vi "MotorSpeedv3.vi"(6 "MotrSpdInfo":T1={"TrgtCounts"=0, "Accel?"=FALSE, "CurrCounts"=0.0, "SlowRng"=572.75, "MinPwr"=572.75} {"MinPwr" format="%#_13g"; "SlowRng" format="%#_13g"}, 7 "MaxPwr":dbl, 8 "RightSpdIn":dbl, 10 "FirstTime?":bool, 11 "LeftSpdIn":dbl) -> (0 "RightSpdOut":dbl, 3 "LeftSpdOut":dbl)   [LabVIEW 2017]
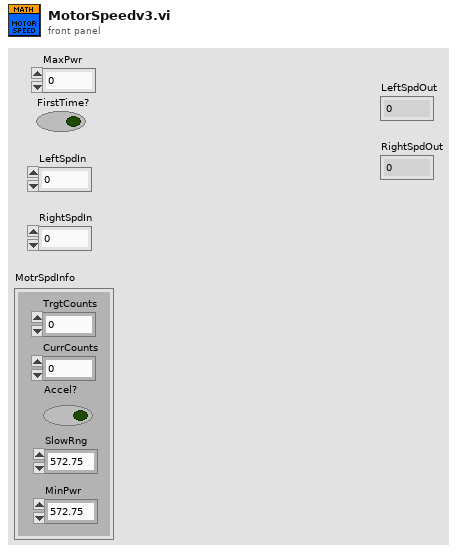
[diagram p1: front panel]
types:
  T1 = cluster{"TrgtCounts":i32, "Accel?":bool, "CurrCounts":dbl, "SlowRng":dbl, "MinPwr":dbl}
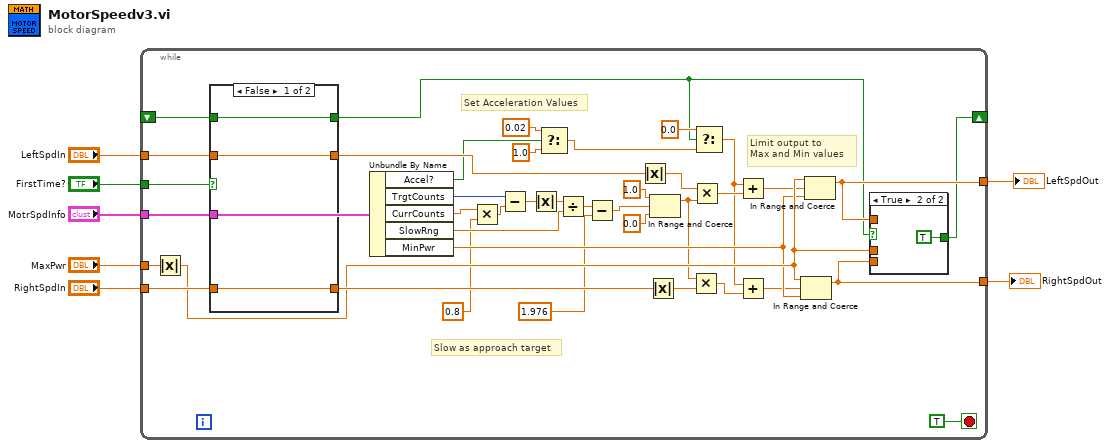
[diagram p0: block diagram]
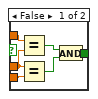
[diagram p2: hidden frame]
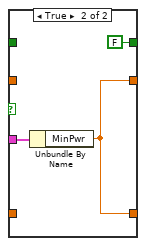
[diagram p3: hidden frame]
diagram:
  n1 = while {
    tunnel: [w47] -> w7
    tunnel: "LeftSpdIn" -> [w43]
    tunnel: "RightSpdIn" -> [w41]
    tunnel: [w46] -> w4
    tunnel: "MotrSpdInfo" -> [w37]
    shift-right: [w45] -> _
    shift-left: _ -> [w38]
    tunnel: "MaxPwr" -> [w36]
    tunnel: "FirstTime?" -> [w39]
    stop <- TRUE stop-if-true
    # "Limit output to\nMax and Min values"
    # "Slow as approach target"
    # "Set Acceleration Values"
    n2 = Absolute Value(x=w36) -> (abs(x)=w35:dbl)
    n3 = case shown="False" w39 {
      tunnel: w43 -> [w57 _]
      tunnel: [w57 w60] -> w42
      tunnel: w41 -> [w56 _]
      tunnel: [w56 w60] -> w40
      tunnel: w38 -> [w55 _]
      tunnel: [w55 FALSE] -> w16
      tunnel: w37 -> [_ w59]
      frame False {
      }
      frame True {
        n4 = Unbundle By Name(w59) -> ("MinPwr"=w60:dbl)
      }
    }
    n5 = Unbundle By Name(w37) -> ("Accel?"=w27:bool, "TrgtCounts"=w29:i32, "CurrCounts"=w13:dbl, "SlowRng"=w28:dbl, "MinPwr"=w24:dbl)
    n6 = Multiply(x=w13, y=0.8 ("f")) -> (x*y=w12:dbl)
    n7 = Subtract(x=w29, y=w12) -> (x-y=w31:dbl)
    n8 = Absolute Value(x=w31) -> (abs(x)=w30:dbl)
    n9 = Select(t=0.02, s=w27, f=1.0) -> (s? t:f=w19:dbl)
    n10 = Divide(x=w30, y=w28) -> (x/y=w10:dbl)
    n11 = Subtract(x=w10, y=1.976) -> (x-y=w9:dbl)
    n12 = Absolute Value(x=w42) -> (abs(x)=w32:dbl)
    n13 = Absolute Value(x=w40) -> (abs(x)=w15:dbl)
    n14 = In Range and Coerce(upper limit=1.0 ("f"), x=w9, lower limit=0.0 ("f")) -> (coerced(x)=w14:dbl)  [unwired: 1 out]
    n15 = Multiply(x=w14, y=w15) -> (x*y=w22:dbl)
    n16 = Multiply(x=w32, y=w14) -> (x*y=w25:dbl)
    n17 = Select(t=0.0, s=w16, f=w19) -> (s? t:f=w18:dbl)
    n18 = Add(x=w18, y=w25) -> (x+y=w26:dbl)
    n19 = Add(x=w18, y=w22) -> (x+y=w23:dbl)
    n20 = In Range and Coerce(upper limit=w35, x=w23, lower limit=w24) -> (coerced(x)=w46:dbl)  [unwired: 1 out]
    n21 = In Range and Coerce(upper limit=w35, x=w26, lower limit=w24) -> (coerced(x)=w47:dbl)  [unwired: 1 out]
    n22 = case shown="True" w16 {
      tunnel: w47 -> [w53 _]
      tunnel: w46 -> [w52 _]
      tunnel: [w51 TRUE] -> w45
      tunnel: w35 -> [w50 _]
      frame False {
        n23 = Equal?(x=w53, y=w50) -> (x = y?=w49:bool)
        n24 = Equal?(x=w50, y=w52) -> (x = y?=w48:bool)
        n25 = And(x=w49, y=w48) -> (x .and. y?=w51:bool)
      }
      frame True {
      }
    }
  }
  "LeftSpdOut" <- w7
  "RightSpdOut" <- w4
